vi "nejistoty.vi"() -> ()   [LabVIEW 2022 SP3]
panel:
  out "Nejistota typu A":dbl
  in  "Array":dbl[](array[numeric])
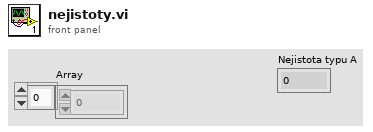
[diagram p1: front panel]
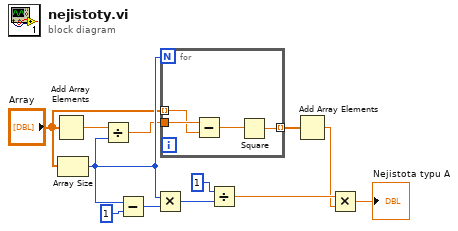
[diagram p0: block diagram]
diagram:
  n1 = Add Array Elements(numeric array="Array") -> (sum=w7:dbl)
  n2 = Array Size(array="Array") -> (size(s)=w6:i32)
  n3 = Divide(x=w7, y=w6) -> (x/y=w5:dbl)
  n4 = Subtract(x=w6, y=1) -> (x-y=w10:i32)
  n5 = Multiply(x=w6, y=w10) -> (x*y=w9:i32)
  n6 = for {
    N: w6 -> [_]
    tunnel: w5 -> [w16]
    tunnel: "Array" -> [w15] mode=indexing
    tunnel: [w13] -> w3 mode=indexing
    n7 = Subtract(x=w16, y=w15) -> (x-y=w14:dbl)
    n8 = Square(x=w14) -> (x^2=w13:dbl)
  }
  n9 = Divide(x=1, y=w9) -> (x/y=w8:dbl)
  n10 = Add Array Elements(numeric array=w3) -> (sum=w2:dbl)
  n11 = Multiply(x=w8, y=w2) -> (x*y=→"Nejistota typu A":dbl)
